vi "Station.SwButtons.Fglb.vi"(1 "action (get)":T2) -> (2 "Buttons":T1)   [LabVIEW 2016]
uses:
  Station.SwButtons.Fglb.Action.ctl
  Station.Buttons.ctl
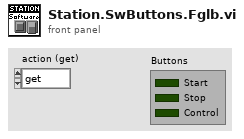
[diagram p1: front panel]
types:
  T1 = typedef "Station.Buttons.ctl" = cluster{"Start":bool, "Stop":bool, "Control":bool}
  T2 = typedef "Station.SwButtons.Fglb.Action.ctl" = enum16{"get", "start", "stop", "control"}
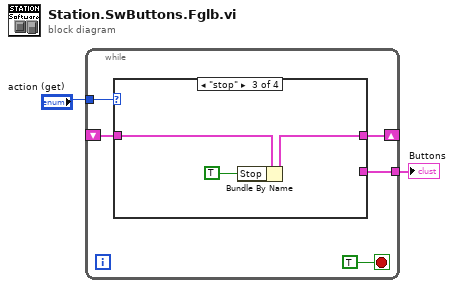
[diagram p0: block diagram]
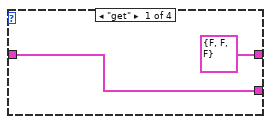
[diagram p2: hidden frame]
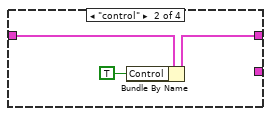
[diagram p3: hidden frame]
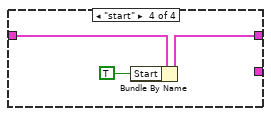
[diagram p4: hidden frame]
diagram:
  n1 = while {
    tunnel: "action (get)" -> [w7]
    shift-right: [w6] -> _
    shift-left: _ -> [w5]
    tunnel: [w3] -> w1
    stop <- TRUE stop-if-true
    n2 = case shown="\"stop\"" w7 {
      tunnel: [T1 {"Start"=FALSE, "Stop"=FALSE, "Control"=FALSE} ("ButtonSw") w10 w13 w16] -> w6
      tunnel: w5 -> [w9 w11 w14 w17]
      tunnel: [w9 _ _ _] -> w3
      frame "get" {
      }
      frame "control" {
        n3 = Bundle By Name(cluster=w11, "Control"=TRUE ("Start")) -> (w10:T1)
      }
      frame "stop" {
        n4 = Bundle By Name(cluster=w14, "Stop"=TRUE ("Start")) -> (w13:T1)
      }
      frame "start" {
        n5 = Bundle By Name(cluster=w17, "Start"=TRUE) -> (w16:T1)
      }
    }
  }
  "Buttons" <- w1
